vi "Is VI Running Top Level.vi"(10 "Error in":errorcluster caption="Error in (no error)", 11 "VI to Check":refnum<vi>) -> (2 "Error out":errorcluster, 3 "Top Level":bool)   [LabVIEW 2018]
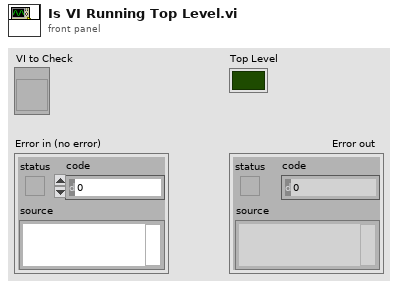
[diagram p1: front panel]
types:
  T1 = enum32{"Bad", "Idle", "Run top level", "Running"}
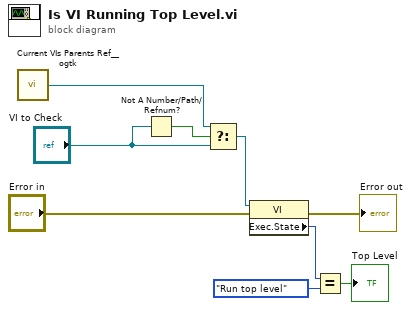
[diagram p0: block diagram]
diagram:
  n1 = call <userlib>:"Current VIs Parents Ref__ogtk.vi"() -> ("Calling VI's Reference"=w3:refnum<vi>)  [unwired: 2 in]
  n2 = Not A Number/Path/Refnum?(number/path/refnum="VI to Check") -> (NaN/Path/Refnum?=w4:bool)
  n3 = Select(t=w3, s=w4, f="VI to Check") -> (s? t:f=w2:refnum<vi>)
  n4 = property class="VI"(reference=w2, error in="Error in") -> (error out=→"Error out":errorcluster, "Exec.State"=w7:T1)  [unwired: 1 out]
  n5 = Equal?(x=w7, y=T1."Run top level") -> (x = y?=→"Top Level":bool)
